vi "CAN-LIN Raw Bus Capture_client.vi"() -> ()   [LabVIEW 2025]
uses:
  can-lin/CAN-LIN Raw Bus Capture UI/OOB gRPC Client/RPC Messages/hwval_BoolRequest.ctl
  can-lin/CAN-LIN Raw Bus Capture UI/OOB gRPC Client/RPC Messages/hwval_ExportRequest.ctl
  can-lin/CAN-LIN Raw Bus Capture UI/OOB gRPC Client/RPC Messages/hwval_GenericRequest.ctl
  can-lin/CAN-LIN Raw Bus Capture UI/OOB gRPC Client/OOB gRPC Client.lvlib
panel:
  out "error out":errorcluster
  in  "Address":string
  out "Address":string
  in  "stop":bool
  in  "Export":bool
  in  "Export File Type":string(combo)="RAW"
  in  "STOP":bool
  in  "PauseResume":bool caption="Pause"
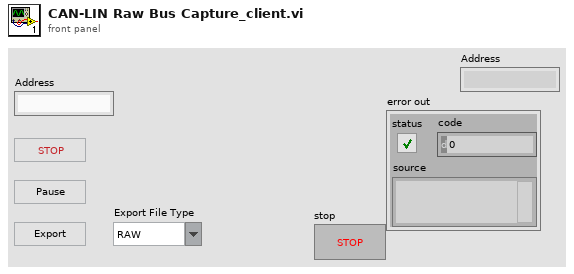
[diagram p1: front panel]
types:
  T1 = typedef "grpc-lvsupport-release.lvlib/grpcId.ctl" = u64
  T2 = typedef "OOB gRPC Client.lvlib/hwval_BoolRequest.ctl" = cluster{"BooleanData":bool}
  T3 = typedef "OOB gRPC Client.lvlib/hwval_ExportRequest.ctl" = cluster{"FileType":string}
  T4 = typedef "OOB gRPC Client.lvlib/hwval_GenericRequest.ctl" = cluster{"Command":string, "Payload":u8[]}
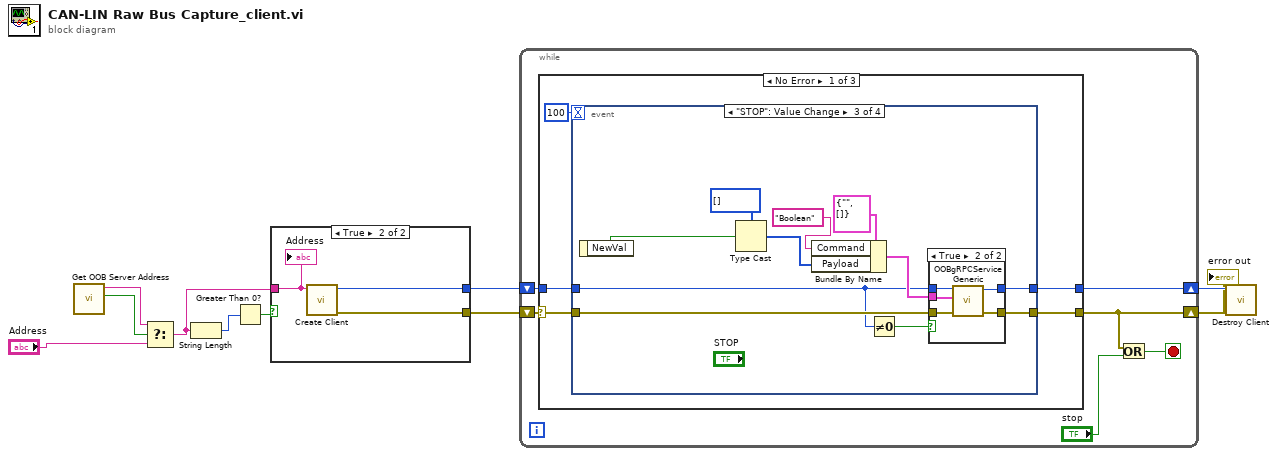
[diagram p0: block diagram]
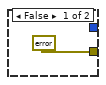
[diagram p2: hidden frame]
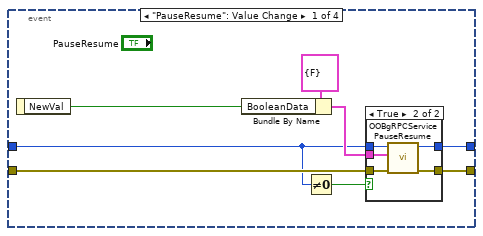
[diagram p3: hidden frame]
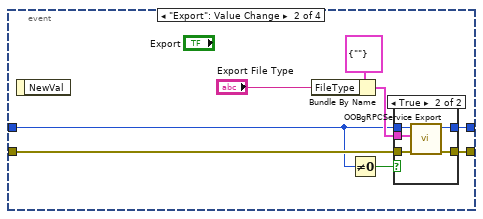
[diagram p5: hidden frame]
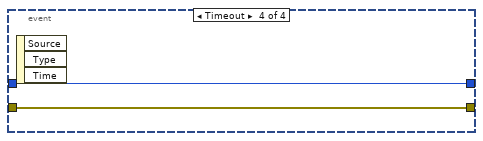
[diagram p8: hidden frame]
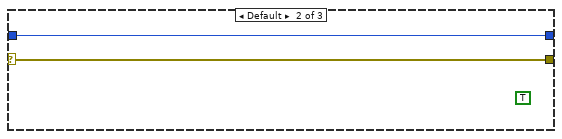
[diagram p9: hidden frame]
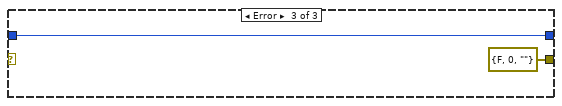
[diagram p10: hidden frame]
diagram:
  n1 = call "Get OOB Server Address.vi"() -> ("Boolean"=w7:bool, "String"=w6:string)  [unwired: 10 in]
  n2 = Select(t=w6, s=w7, f="Address") -> (s? t:f=w4:string)
  n3 = String Length(string=w4) -> (length=w2:i32)
  n4 = Greater Than 0?(x=w2) -> (x > 0?=w3:bool)
  n5 = case shown="True" w3 {
    tunnel: w4 -> [_ w14]
    tunnel: [_ w13] -> w10
    tunnel: [errorcluster {"status"=TRUE, "code"=-1, "source"="Set  a valid Server Port"} ("error out") w12] -> w9
    frame False {
    }
    frame True {
      n6 = call "Create Client.vi"("address"=w14) -> ("error out"=w12:errorcluster, "gRPC ID Out"=w13:T1)  [unwired: 9 in]
      "Address" <- w14
    }
  }
  n7 = while {
    shift-right: [w15] -> w1
    shift-left: w9 -> [w20]
    shift-right: [w18] -> w8
    shift-left: w10 -> [w19]
    stop <- w17 stop-if-true
    n8 = case shown="No Error" w20 {
      selector: w20 -> [w24 w76 _]
      tunnel: [w25 w76 errorcluster {"status"=FALSE, "code"=0, "source"=""} ("error IO")] -> w15
      tunnel: w19 -> [w23 w77 w78]
      tunnel: [w22 w77 w78] -> w18
      frame No Error {
        n9 = event shown="[2] \"STOP\": Value Change" {
          selector: _ -> [_ _ _ _]
          dyn-events: _ -> [_ _ _ _]
          timeout: 100 -> [_ _ _ _]
          tunnel: [w32 w47 w65 w74] -> w25
          tunnel: w24 -> [w31 w46 w64 w74]
          tunnel: w23 -> [w26 w42 w61 w75]
          tunnel: [w33 w48 w66 w75] -> w22
          event "PauseResume": Value Change {
            n10 = event-data() -> ("NewVal"=w28:bool)  [unwired: 1 in]
            n11 = Bundle By Name(cluster=T2 {"BooleanData"=FALSE} ("Request Data"), "BooleanData"=w28) -> (w29:T2)
            n12 = Not Equal To 0?(x=w26) -> (x != 0?=w27:bool)
            n13 = case shown="True" w27 {
              tunnel: [w35 w40] -> w33
              tunnel: [w34 w39] -> w32
              tunnel: w26 -> [w35 w38]
              tunnel: w31 -> [w34 w37]
              tunnel: w29 -> [_ w36]
              frame False {
              }
              frame True {
                n14 = call "OOBgRPCService PauseResume.vi"("error in"=w37, "Request Data"=w36, "gRPC ID"=w38) -> ("error out"=w39:errorcluster, "gRPC ID out"=w40:T1)  [unwired: 6 in, 1 out]
              }
            }
          }
          event "Export": Value Change {
            n15 = event-data() -> ()  [unwired: 1 in, 1 out]
            n16 = Bundle By Name(cluster=T3 {"FileType"=""} ("Request Data"), "FileType"="Export File Type") -> (w44:T3)
            n17 = Not Equal To 0?(x=w42) -> (x != 0?=w43:bool)
            n18 = case shown="True" w43 {
              tunnel: [w50 w55] -> w48
              tunnel: [w49 w54] -> w47
              tunnel: w42 -> [w50 w53]
              tunnel: w46 -> [w49 w52]
              tunnel: w44 -> [_ w51]
              frame False {
              }
              frame True {
                n19 = call "OOBgRPCService Export.vi"("error in"=w52, "Request Data"=w51, "gRPC ID"=w53) -> ("error out"=w54:errorcluster, "gRPC ID out"=w55:T1)  [unwired: 6 in, 1 out]
              }
            }
          }
          event "STOP": Value Change {
            n20 = event-data() -> ("NewVal"=w58:bool)  [unwired: 1 in]
            n21 = Type Cast(type=u8[] [] ("Payload"), x=w58) -> (*(type *) &x=w57:u8[])
            n22 = Bundle By Name(cluster=T4 {"Command"="", "Payload"=[]} ("Request Data"), "Command"="Boolean", "Payload"=w57) -> (w63:T4)
            n23 = Not Equal To 0?(x=w61) -> (x != 0?=w62:bool)
            n24 = case shown="True" w62 {
              tunnel: [w68 w72] -> w66
              tunnel: [w67 w71] -> w65
              tunnel: w61 -> [w68 w73]
              tunnel: w64 -> [w67 w70]
              tunnel: w63 -> [_ w69]
              frame False {
              }
              frame True {
                n25 = call "OOBgRPCService Generic.vi"("error in"=w70, "Request Data"=w69, "gRPC ID"=w73) -> ("error out"=w71:errorcluster, "gRPC ID out"=w72:T1)  [unwired: 6 in, 1 out]
              }
            }
          }
          event Timeout {
            n26 = event-data() -> ()  [unwired: 1 in, 3 out]
          }
        }
      }
      frame Default {
        (unwired) TRUE
      }
      frame Error {
      }
    }
    n27 = Or(x=w15, y="stop") -> (x .or. y?=w17:bool)
  }
  "error out" <- w1
  n28 = call "Destroy Client.vi"("gRPC ID"=w8) -> ()  [unwired: 10 in, 1 out]
